vi "Function Set.vi"(6 "chip select (1st chip)":enum16{"1st chip", "2nd chip"}(ring), 8 "error in (no error)":errorcluster, 10 "font configuration (5x8 & 2 lines)":T1(ring), 11 "HD44780 in":refnum<class "HD44780.lvclass">) -> (0 "error out":errorcluster, 3 "HD44780 out":refnum<class "HD44780.lvclass">)   [LabVIEW 2017, in "HD44780.lvclass"]
uses:
  HD44780.lvclass
  HD44780.lvclass/HD44780.ctl
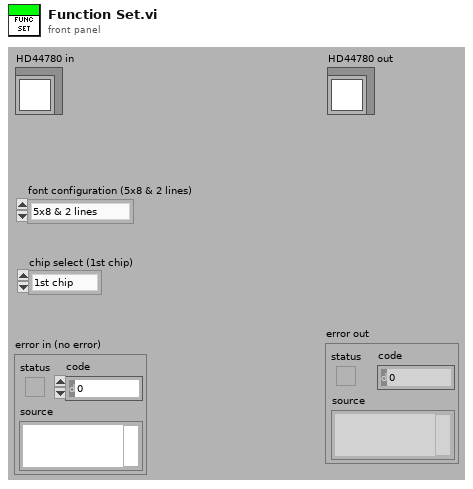
[diagram p1: front panel]
types:
  T1 = enum8{"5x8 & 2 lines", "5x10 & 1 line", "5x8 & 1 line"}
  T2 = typedef "HD44780 Common.lvlib/cluster of class private data.ctl" = cluster{"FPGA VI Reference":refnum<k20>, "device index":i8, "screen size":T3, "font size":T4, "auto wrap":bool, "alignment":T5, "number of line":T6, "shift 0":i8, "entry mode 0":T7, "shift 1":i8, "entry mode 1":T7}
  T3 = typedef "HD44780 Common.lvlib/screen size.ctl" = enum8{"8x1", "8x2", "12x4", "16x1", "16x2", "16x4", "20x1", "20x2", "20x4", "24x1", "24x2", "40x2", "40x4"}
  T4 = typedef "HD44780 Common.lvlib/font size.ctl" = enum8{"5x8", "5x10"}
  T5 = typedef "HD44780 Common.lvlib/alignment.ctl" = enum16{"None", "Left", "Center", "Right"}
  T6 = typedef "HD44780 Common.lvlib/line number.ctl" = enum8{"1 line", "2 lines"}
  T7 = typedef "HD44780 Common.lvlib/entry mode.ctl" = enum8{"increment & no shift", "increment & shift", "decrement & no shift", "decrement & shift"}
  T8 = cluster{"FPGA VI Reference":refnum<k20>, "device index":i8, "screen size":enum8{"8x1", "8x2", "12x4", "16x1", "16x2", "16x4", "20x1", "20x2", "20x4", "24x1", "24x2", "40x2", "40x4"}, "font size":enum8{"5x8", "5x10"}, "auto wrap":bool, "alignment":enum16{"None", "Left", "Center", "Right"}, "number of line":enum8{"1 line", "2 lines"}, "shift 0":i8, "entry mode 0":enum8{"increment & no shift", "increment & shift", "decrement & no shift", "decrement & shift"}, "shift 1":i8, "entry mode 1":enum8{"increment & no shift", "increment & shift", "decrement & no shift", "decrement & shift"}}
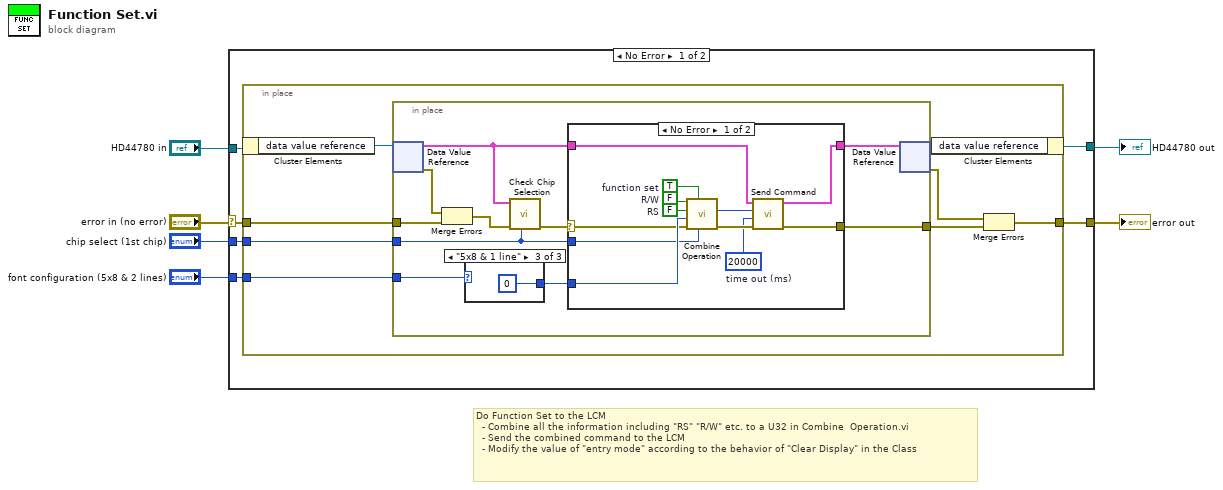
[diagram p0: block diagram]
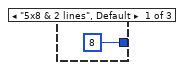
[diagram p2: hidden frame]
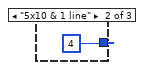
[diagram p3: hidden frame]
diagram:
  # "Do Function Set to the LCM\n  - Combine all the information including \"RS\" \"R/W\" etc. to a U32 in Combine  Operation.vi \n  - Send the combined command to the LCM\n  - Modify the value of \"entry mode\" according to the behavior of \"Clear Display\" in the Class"
  n1 = case shown="No Error" "error in (no error)" {
    selector: "error in (no error)" -> [w7 w48]
    tunnel: [w12 w48] -> w6
    tunnel: "font configuration (5x8 & 2 lines)" -> [w11 _]
    tunnel: "chip select (1st chip)" -> [w10 _]
    tunnel: "HD44780 in" -> [w9 w49]
    tunnel: [w8 w49] -> w1
    frame No Error {
      n2 = in-place {
        in-place-border: [w16] -> w12
        in-place-border: w11 -> [w20]
        in-place-border: w10 -> [w19]
        in-place-border: w7 -> [w13]
        n3 = in-place-cluster #1(w9) -> ("data value reference"=w18:refnum<data-value>)
        n4 = in-place {
          in-place-border: [w30] -> w14
          in-place-border: w20 -> [w23]
          in-place-border: w19 -> [w21]
          in-place-border: w13 -> [w27]
          n5 = in-place-dvr #2(w18) -> (w29:T2, w28:errorcluster)
          n6 = Merge Errors(w28, w27) -> (w26:errorcluster)
          n7 = case shown="\"5x8 & 1 line\"" w23 {
            tunnel: [u8 8 u8 4 u8 0] -> w22
            frame "5x8 & 2 lines", Default {
            }
            frame "5x10 & 1 line" {
            }
            frame "5x8 & 1 line" {
            }
          }
          n8 = call "Check Chip Selection.vi"("chip select"=w21, "error in (no error)"=w26, "cluster of private data in"=w29) -> ("error out"=w25:errorcluster)  [unwired: 7 in, 1 out]
          n9 = case shown="No Error" w25 {
            selector: w25 -> [w35 w47]
            tunnel: [w45 w47] -> w30
            tunnel: w29 -> [w44 w46]
            tunnel: [w38 w46] -> w24
            tunnel: w22 -> [w37 _]
            tunnel: w21 -> [w36 _]
            frame No Error {
              w34 = u32 20000  # time out (ms)
              w39 = FALSE  # RS
              w42 = TRUE  # function set
              w43 = FALSE  # R/W
              n10 = call "Combine Operation.vi"("chip select  (1st chip)"=w36, "function set (F)"=w42, "error in (no error)"=w35, "cmd/data"=w37, "RS"=w39, "R/W"=w43) -> ("error out"=w41:errorcluster, "output"=w40:u32)  [unwired: 4 in]
              n11 = call "Send Command.vi"("error in (no error)"=w41, "time out? (ms)"=w34, "operation"=w40, "cluster of private data in"=w44) -> ("error out"=w45:errorcluster, "cluster of private data out"=w38:T8)  [unwired: 5 in, 1 out]
            }
            frame Error {
            }
          }
          n12 = in-place-dvr #2(w24) -> (w17:refnum<data-value>, w15:errorcluster)
        }
        n13 = in-place-cluster #1("data value reference"=w17) -> (w8:refnum<class "HD44780.lvclass">)
        n14 = Merge Errors(w15, w14) -> (w16:errorcluster)
      }
    }
    frame Error {
    }
  }
  "HD44780 out" <- w1
  "error out" <- w6
